vi "Mapping v10.2.0.vi"(5 "Simulate Spectra":bool, 7 "Simulate Drive":bool, 11 "Input Parameters":T7={"CCD3000 Connection"={"Comm Interface"=1, "BUS"=0, "Address"=5, "Com Port"=1}, "Drive Connection Settings"={"Objective GPIB-Port"=4, "Stage GPIB-Port"=4, "Drive Selector"=0, "Drive Velocity (V/s)"=5.0}, "ITC503 Current Values"={"ITC503 Heater"=0.0, "ITC503 Temperature"=0.0, "ITC503 P"=0.0, "ITC503 I"=0.0, "ITC503 D"=0.0, "ITC503 Setpoint"=0.0, "ITC503 Gradient"=0.0, "ITC503 Heater Auto"=FALSE, "ITC503 PID Auto"=FALSE}, "Wavelengths (nm)"=[], "Drive Current Values"={"Voltages"={"Drive X Voltage"=0.0, "Drive Y Voltage"=0.0, "Drive Z Voltage"=0.0}, "Position"={"Drive X Position"=0.0, "Drive Y Position"=0.0, "Drive Z Position"=0.0}}, "iHR Current Values"={"iHR 550 Front Entrance"=0.0, "iHR550 Side Exit"=0.0, "iHR550 Wavelength"=897.9988, "iHR550 Exit Mirror"=2, "iHR550 Grating"="1", "Grating Index"=1}, "Spectra Settings"={"Integration Time"=1.0, "Repetitions"=1, "Mapping Spectra"=TRUE}, "CCD3500 Temperature"=0.0, "Simulate Drive"=FALSE, "Simulate Spectra"=FALSE} {"CCD3500 Temperature" min=10.0 max=160.0 step=0.1 format="%.1f"; "Spectra Settings"."Repetitions" min=1 max=100 step=1; "Spectra Settings"."Integration Time" min=0.5 max=6000.0 step=1.0 format="%.1f"; "iHR Current Values"."iHR550 Exit Mirror" items=["EntranceMirror", "ExitMirror", "Front", "Side"]; "Drive Current Values"."Position"."Drive Z Position" min=-273.0 max=300000.0 step=0.0001 format="%.1f"; "Drive Current Values"."Position"."Drive Y Position" min=-273.0 max=300000.0 step=0.0001 format="%.1f"; "Drive Current Values"."Position"."Drive X Position" min=-273.0 max=300000.0 step=0.0001 format="%.1f"; "Drive Current Values"."Voltages"."Drive Z Voltage" min=-273.0 max=300000.0 step=0.0001 format="%.1f"; "Drive Current Values"."Voltages"."Drive Y Voltage" min=-273.0 max=300000.0 step=0.0001 format="%.1f"; "Drive Current Values"."Voltages"."Drive X Voltage" min=-273.0 max=300000.0 step=0.0001 format="%.1f"; "ITC503 Current Values"."ITC503 Gradient" format="%.2f"; "ITC503 Current Values"."ITC503 Setpoint" min=-273.0 max=300000.0 step=0.0001 format="%.1f"; "ITC503 Current Values"."ITC503 I" format="%_1f"; "ITC503 Current Values"."ITC503 P" format="%_1f"; "ITC503 Current Values"."ITC503 Temperature" min=0.0 max=1645.0 step=1e-05 format="%.2f"; "ITC503 Current Values"."ITC503 Heater" min=0.0 max=100.0 step=0.01 scale=0.0..100.0; "Drive Connection Settings"."Drive Velocity (V/s)" min=10.0 max=160.0 step=0.1 format="%.1f"; "Drive Connection Settings"."Drive Selector" items=["Obj.", "Stage"]; "Drive Connection Settings"."Stage GPIB-Port" min=1 max=20 step=1 format="%#.0f"; "Drive Connection Settings"."Objective GPIB-Port" min=1 max=20 step=1 format="%#.0f"; "CCD3000 Connection"."Comm Interface" items=["RS 232", "GPIB"]}) -> ()   [LabVIEW 2010]
uses:
  ESA-C/TypeDefs/ESA-C Connection Settings.ctl
  TypeDefs/Mapping Spectra Params.ctl
  TypeDefs/Mapping Drive Params.ctl
  ESA-C/TypeDefs/ESA-C Set Positions.ctl
  ESA-C/TypeDefs/ESA-C Current Values.ctl
  iHR550/TypeDefs/iHR Current Values.ctl
  ITC503/TypeDefs/ITC503 Current Values.ctl
  drivers/Horiba Spectrum One 3000V/Lib/CCD_command.llb/Comm Params.ctl
  <vilib>/Utility/miscctls.llb/LVPointTypeDef.ctl
panel:
  in  "Save Map":bool
  out "Filename":string
  out "Full Data":dbl[][](array[numeric])
  in  "CCD3000 Current Rep.":string="0/0"
  in  "CCD3500V Connection":T8={"Comm Interface"=1, "BUS"=0, "Address"=5, "Com Port"=0}
  out "Live Data":dbl[][](array[numeric])
  in  "ITC503 Current Values":T3 {"ITC503 Gradient" format="%.2f"; "ITC503 Setpoint" min=-273.0 max=300000.0 step=0.0001 format="%.1f"; "ITC503 I" format="%_1f"; "ITC503 P" format="%_1f"; "ITC503 Temperature" min=0.0 max=1645.0 step=1e-05 format="%.2f"; "ITC503 Heater" min=0.0 max=100.0 step=0.01 scale=0.0..100.0}
  in  "iHR Current Values":T5={"iHR 550 Front Entrance"=0.0, "iHR550 Side Exit"=0.0, "iHR550 Wavelength"=897.9988, "iHR550 Exit Mirror"=2, "iHR550 Grating"="1", "Grating Index"=1} {"iHR550 Exit Mirror" items=["EntranceMirror", "ExitMirror", "Front", "Side"]}
  in  "CCD3500 Temperature":dbl caption="Temp. (°C)" min=10.0 max=160.0 step=0.1 format="%.1f"
  in  "Wavelengths (nm)":dbl[](array[numeric])
  in  "Spectra Params":T6={"Integration Time"=10.0, "Repetitions"=10, "Mapping Spectra"=TRUE} {"Repetitions" min=1 max=100 step=1; "Integration Time" min=0.5 max=6000.0 step=1.0 format="%.1f"}
  in  "Drive Settings":T2={"Objective GPIB-Port"=4, "Stage GPIB-Port"=4, "Drive Selector"=0, "Drive Velocity (V/s)"=5.0} {"Drive Velocity (V/s)" min=10.0 max=160.0 step=0.1 format="%.1f"; "Drive Selector" items=["Obj.", "Stage"]; "Stage GPIB-Port" min=1 max=20 step=1 format="%#.0f"; "Objective GPIB-Port" min=1 max=20 step=1 format="%#.0f"}
  out "Current Position":T4 {"Position"."Drive Z Position" min=-273.0 max=300000.0 step=0.0001 format="%.1f"; "Position"."Drive Y Position" min=-273.0 max=300000.0 step=0.0001 format="%.1f"; "Position"."Drive X Position" min=-273.0 max=300000.0 step=0.0001 format="%.1f"; "Voltages"."Drive Z Voltage" min=-273.0 max=300000.0 step=0.0001 format="%.1f"; "Voltages"."Drive Y Voltage" min=-273.0 max=300000.0 step=0.0001 format="%.1f"; "Voltages"."Drive X Voltage" min=-273.0 max=300000.0 step=0.0001 format="%.1f"}
  out "Target Position":T9={"Drive X Set"=10.0, "Drive Y Set"=10.0, "Drive Z Set"=10.0} {"Drive X Set" min=10.0 max=160.0 step=0.1 format="%.1f"; "Drive Z Set" min=10.0 max=160.0 step=0.1 format="%.1f"; "Drive Y Set" min=10.0 max=160.0 step=0.1 format="%.1f"}
  out "Progress":u8(slide) max=10 scale=0.0..100.0
  out "Objective Running":bool caption="Obj."
  out "CCD Running":bool caption="CCD"
  in  "Z Position":dbl caption="Z (µm)" min=0.0 max=100.0 step=0.1 format="%.1f"
  in  "Mapping Params":T10={"X Start Position"=0.0, "X Stop Position"=10.0, "Y Start Position"=0.0, "Y Stop Position"=10.0, "Step Size"=1.0} {"Step Size" min=0.1 max=30.0 step=0.1 format="%.1f"; "Y Stop Position" min=0.0 max=30.0 step=0.1 format="%.1f"; "Y Start Position" min=0.0 max=30.0 step=0.1 format="%.1f"; "X Stop Position" min=0.0 max=30.0 step=0.1 format="%.1f"; "X Start Position" min=0.0 max=30.0 step=0.1 format="%.1f"}
  in  "Exit":bool
  out "Measuring":bool
  in  "Start":bool
  # "Spectral"
  # "Spectral / Video Mapping"
  # "Parameters"
  # "GPIB"
  # "Status"
  # "Active"
  # "Target"
  # "Current"
  # "Mapping"
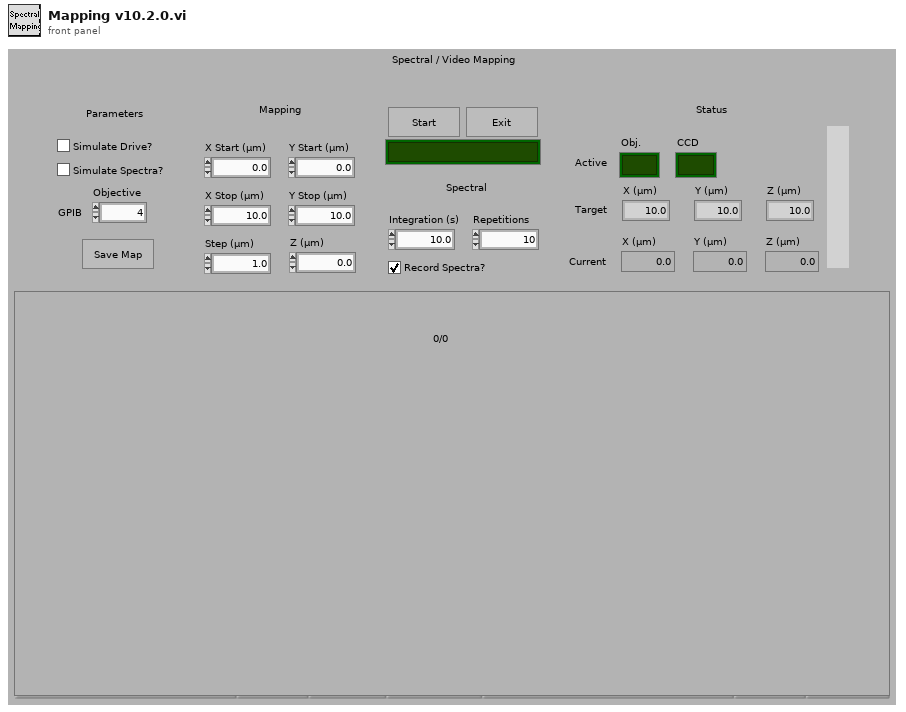
[diagram p1: front panel]
types:
  T1 = typedef "Comm Params.ctl" = cluster{"Comm Interface":u16, "BUS":i16, "Address":i16, "Com Port":i32}
  T2 = typedef "ESA-C Connection Settings.ctl" = cluster{"Objective GPIB-Port":i32, "Stage GPIB-Port":i32, "Drive Selector":u16, "Drive Velocity (V/s)":dbl}
  T3 = typedef "ITC503 Current Values.ctl" = cluster{"ITC503 Heater":dbl, "ITC503 Temperature":dbl, "ITC503 P":dbl, "ITC503 I":dbl, "ITC503 D":dbl, "ITC503 Setpoint":dbl, "ITC503 Gradient":dbl, "ITC503 Heater Auto":bool, "ITC503 PID Auto":bool}
  T4 = typedef "ESA-C Current Values.ctl" = cluster{"Voltages":cluster{"Drive X Voltage":dbl, "Drive Y Voltage":dbl, "Drive Z Voltage":dbl}, "Position":cluster{"Drive X Position":dbl, "Drive Y Position":dbl, "Drive Z Position":dbl}}
  T5 = typedef "iHR Current Values.ctl" = cluster{"iHR 550 Front Entrance":dbl, "iHR550 Side Exit":dbl, "iHR550 Wavelength":dbl, "iHR550 Exit Mirror":i32, "iHR550 Grating":string, "Grating Index":i32}
  T6 = typedef "Mapping Spectra Params.ctl" = cluster{"Integration Time":dbl, "Repetitions":u16, "Mapping Spectra":bool}
  T7 = cluster{"CCD3000 Connection":T1, "Drive Connection Settings":T2, "ITC503 Current Values":T3, "Wavelengths (nm)":dbl[], "Drive Current Values":T4, "iHR Current Values":T5, "Spectra Settings":T6, "CCD3500 Temperature":dbl, "Simulate Drive":bool, "Simulate Spectra":bool}
  T8 = cluster{"Comm Interface":u16, "BUS":i16, "Address":i16, "Com Port":i32}
  T9 = typedef "ESA-C Set Positions.ctl" = cluster{"Drive X Set":dbl, "Drive Y Set":dbl, "Drive Z Set":dbl}
  T10 = typedef "Mapping Drive Params.ctl" = cluster{"X Start Position":dbl, "X Stop Position":dbl, "Y Start Position":dbl, "Y Stop Position":dbl, "Step Size":dbl}
  T11 = cluster{"CCD3000 Connection":T1, "Drive Connection Settings":T2, "ITC503 Current Values":T3, "Wavelengths (nm)":dbl[], "Drive Current Values":T4, "iHR Current Values":T5, "Spectra Settings":T6, "CCD3500 Temperature":dbl, "Simulate Drive 2":bool, "Simulate Spectra 2":bool}
  T12 = typedef "LVPointTypeDef.ctl" = cluster{"Horizontal":i16, "Vertical":i16}
  T13 = typedef "NPC3SG Set Positions.ctl" = cluster{"Drive X Set":dbl, "Drive Y Set":dbl, "Drive Z Set":dbl}
  T14 = cluster{"Intensities":dbl[], "Wavelengths":dbl[]}[]
  T15 = cluster{"Intensities":dbl[], "Wavelengths":dbl[]}
  T16 = enum32{"invalid app kind", "Development System", "Run Time System", "Student Edition", "Embedded LabVIEW", "Evaluation", "Custom"}
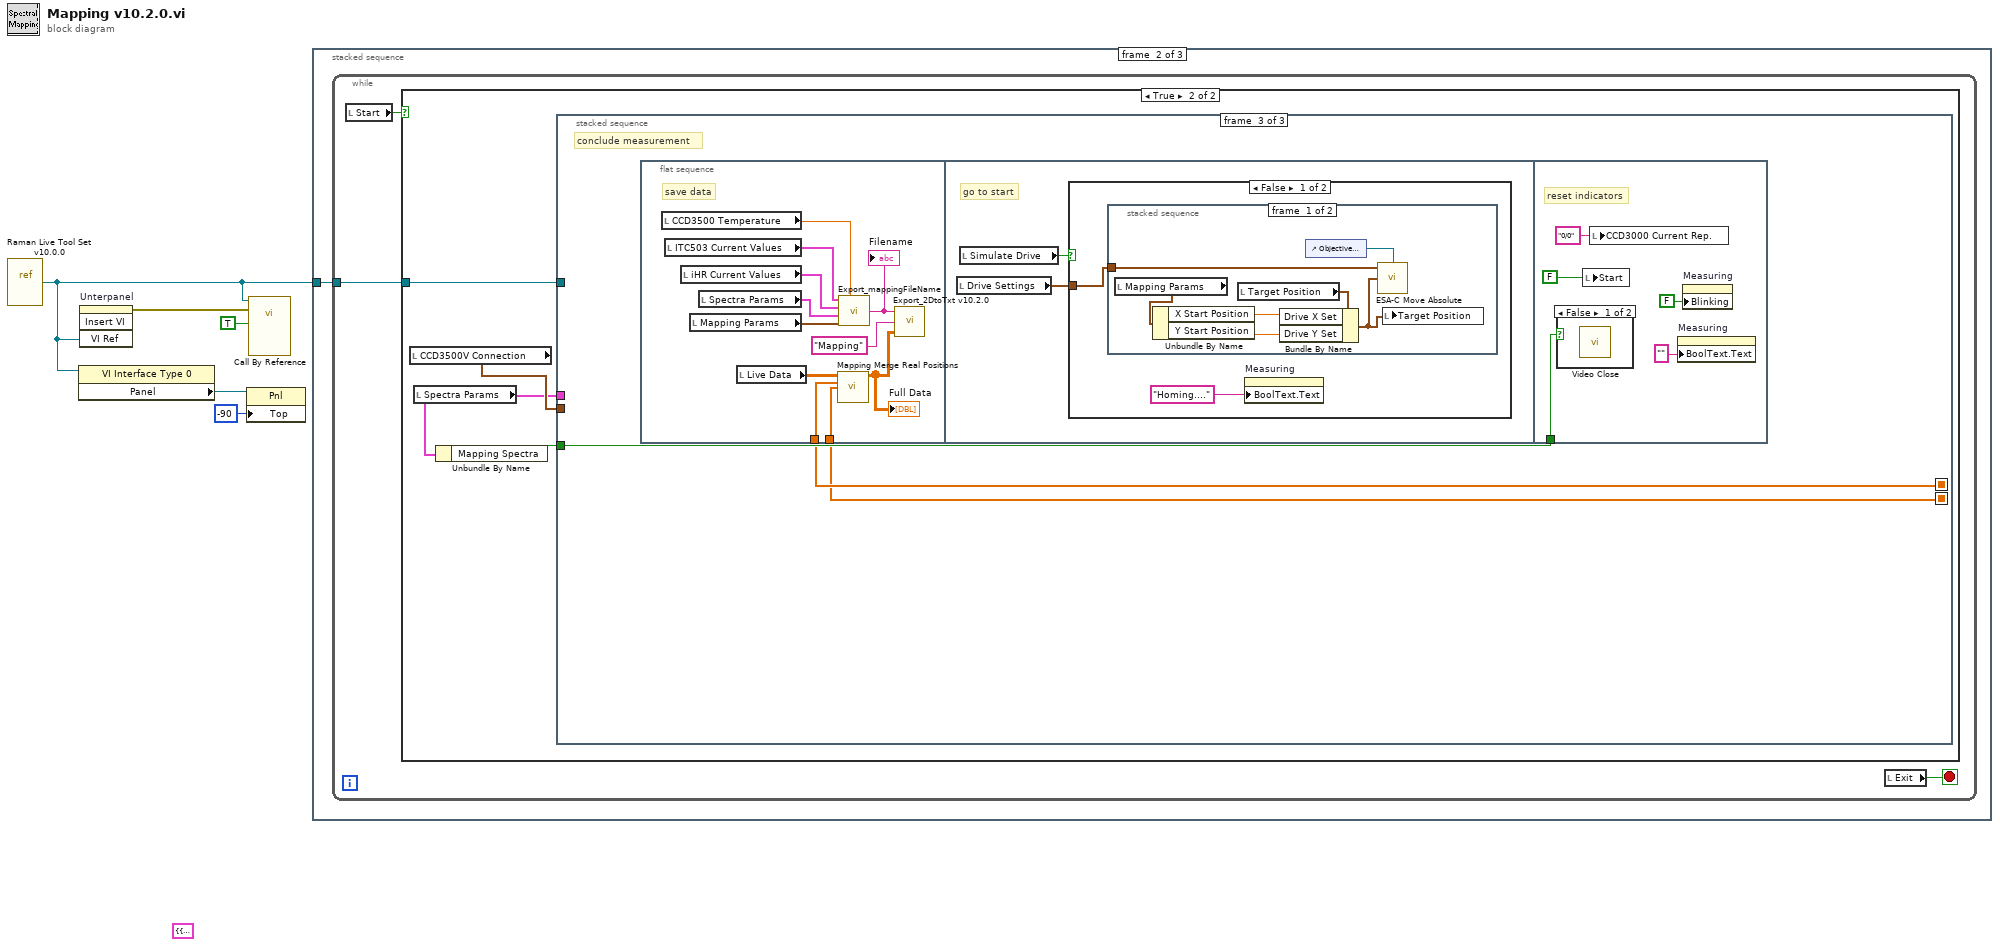
[diagram p0: block diagram]
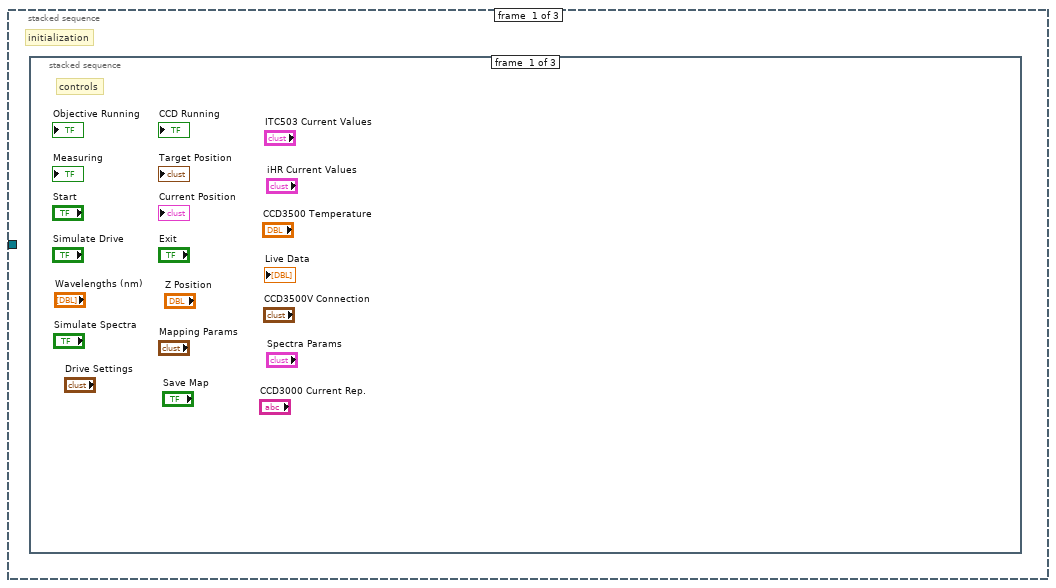
[diagram p2: hidden frame]
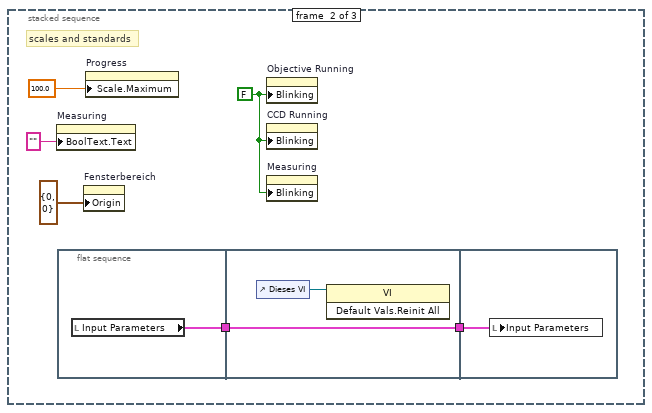
[diagram p3: hidden frame]
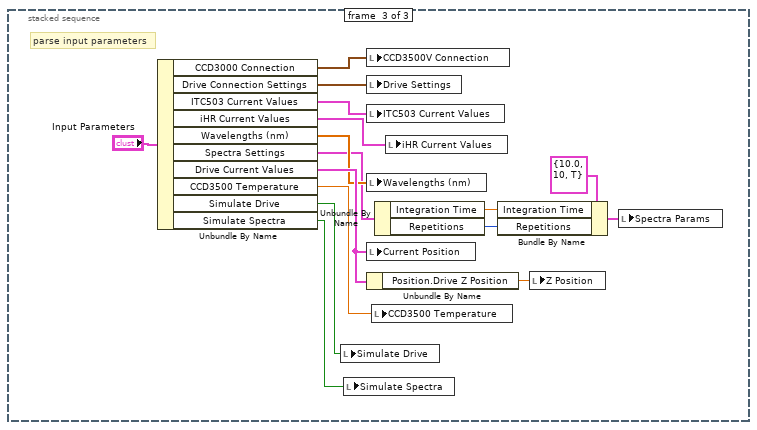
[diagram p4: hidden frame]
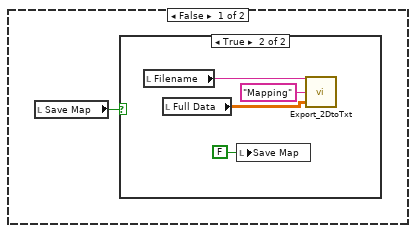
[diagram p5: hidden frame]
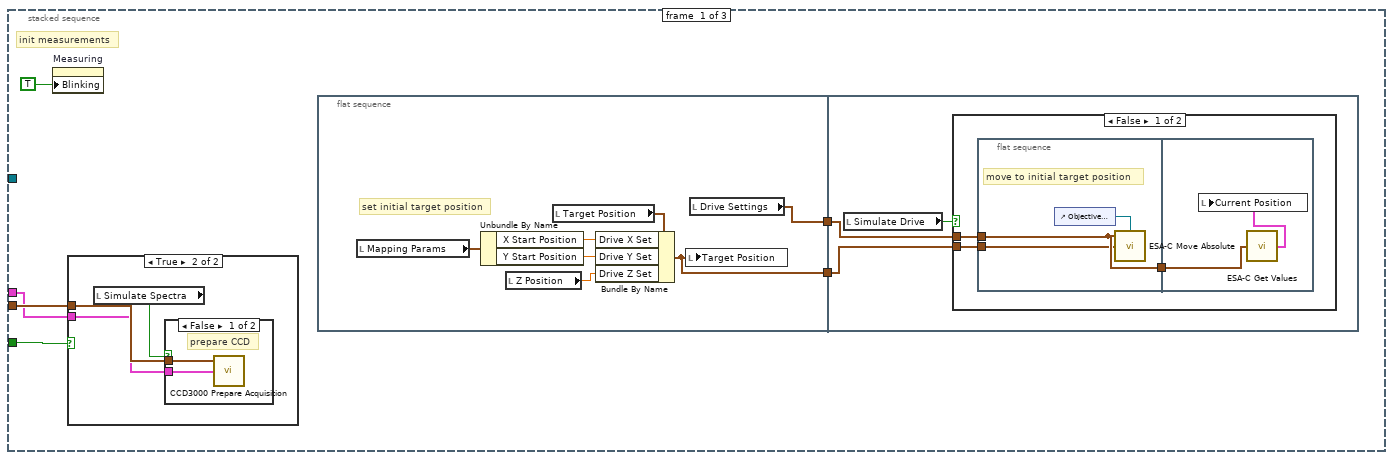
[diagram p7: hidden frame]
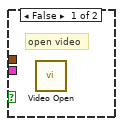
[diagram p9: hidden frame]
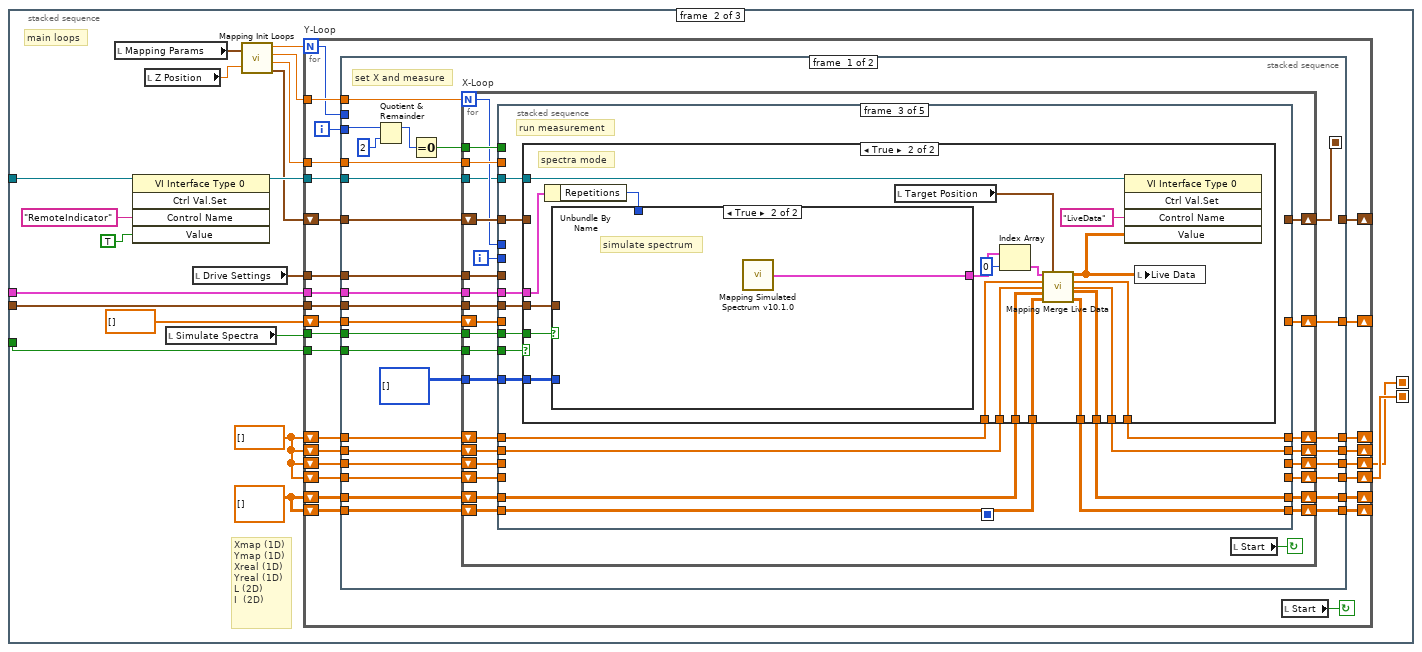
[diagram p11: hidden frame]
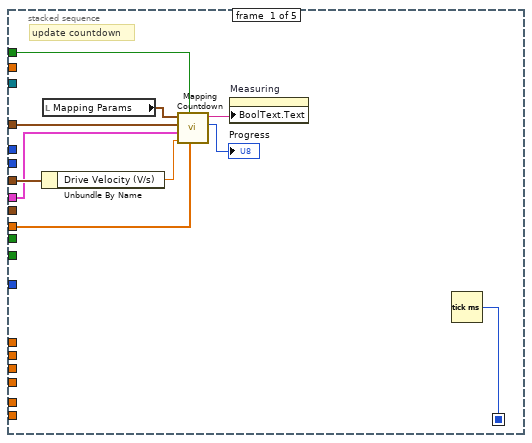
[diagram p12: hidden frame]
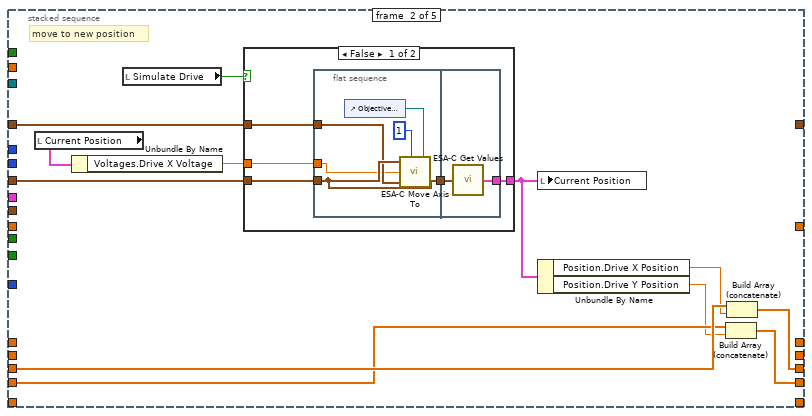
[diagram p13: hidden frame]
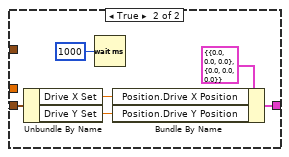
[diagram p14: hidden frame]
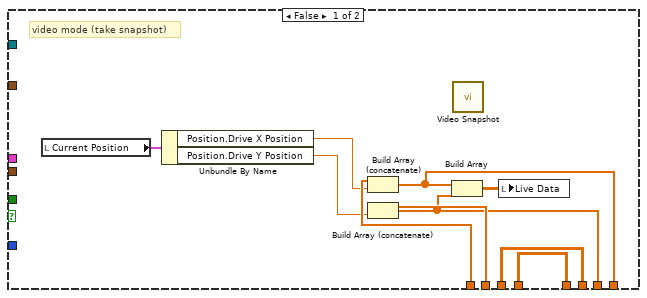
[diagram p15: hidden frame]
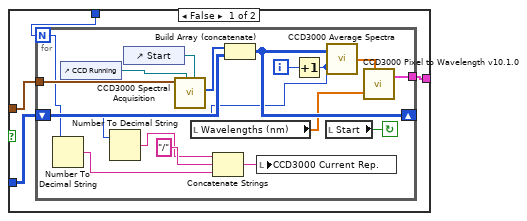
[diagram p16: hidden frame]
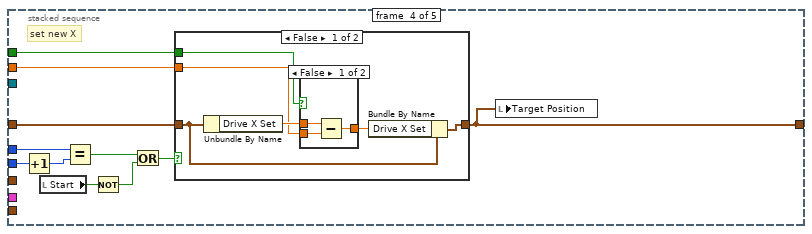
[diagram p17: hidden frame]
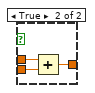
[diagram p18: hidden frame]
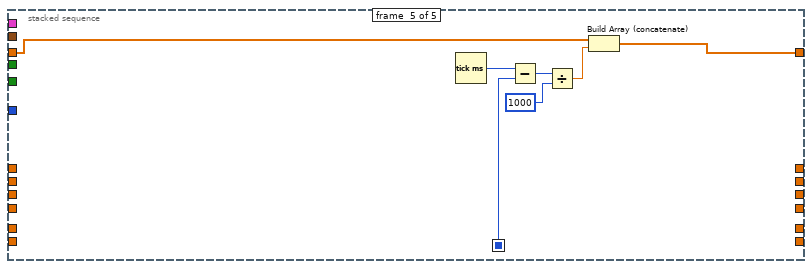
[diagram p20: hidden frame]
diagram:
  (unwired) T11 {"CCD3000 Connection"={"Comm Interface"=1, "BUS"=0, "Address"=5, "Com Port"=1}, "Drive Connection Settings"={"Objective GPIB-Port"=4, "Stage GPIB-Port"=4, "Drive Selector"=0, "Drive Velocity (V/s)"=5.0}, "ITC503 Current Values"={"ITC503 Heater"=0.0, "ITC503 Temperature"=0.0, "ITC503 P"=0.0, "ITC503 I"=0.0, "ITC503 D"=0.0, "ITC503 Setpoint"=0.0, "ITC503 Gradient"=0.0, "ITC503 Heater Auto"=FALSE, "ITC503 PID Auto"=FALSE}, "Wavelengths (nm)"=[], "Drive Current Values"={"Voltages"={"Drive X Voltage"=0.0, "Drive Y Voltage"=0.0, "Drive Z Voltage"=0.0}, "Position"={"Drive X Position"=0.0, "Drive Y Position"=0.0, "Drive Z Position"=0.0}}, "iHR Current Values"={"iHR 550 Front Entrance"=0.0, "iHR550 Side Exit"=0.0, "iHR550 Wavelength"=897.9988, "iHR550 Exit Mirror"=2, "iHR550 Grating"="1", "Grating Index"=1}, "Spectra Settings"={"Integration Time"=1.0, "Repetitions"=1, "Mapping Spectra"=TRUE}, "CCD3500 Temperature"=0.0, "Simulate Drive 2"=FALSE, "Simulate Spectra 2"=FALSE} ("Input Parameters")
  n1 = vi-ref "Raman Live Tool Set v10.0.0.vi"() -> (w3:refnum<vi>)
  n2 = property class="VI Interface Type 0"(reference=w3) -> ("Panel"=w2:refnum<vi>)  [unwired: 1 in, 2 out]
  n3 = invoke on="Unterpanel" class="Unterpanel" method="Insert VI"("VI Ref"=w3) -> (error out=w5:errorcluster)  [unwired: 3 in, 3 out]
  n4 = property class="Pnl"(reference=w2, "Top"=-90 ("Position:Oben")) -> ()  [unwired: 1 in, 2 out]
  n5 = call-by-ref "?"(reference=w3, error in=w5, "RemoteIndicator"=TRUE) -> ()  [unwired: 3 in, 2 out]
  n6 = stacked-sequence {
    tunnel: w3 -> [_ w32 w379]
    frame #0 {
      # "initialization"
      n7 = stacked-sequence {
        frame #0 {
          # "controls"
        }
        frame #1 {
          w9 = FALSE ("Blinkend")
          # "scales and standards"
          n8 = property on="Measuring" class="Bool (strict)"("BoolText.Text"="" ("Boolescher Text.Text")) -> ()  [unwired: 2 in, 2 out]
          n9 = flat-sequence {
            tunnel: [w12] -> w6
            tunnel: [w13] -> w7
            tunnel: w6 -> [w13]
            tunnel: w7 -> [w15]
            frame #0 {
              n10 = local read "Input Parameters"() -> (w12:T7)
            }
            frame #1 {
              n11 = control-ref of="Dieses VI"() -> (w14:refnum<vi>)
              n12 = invoke class="VI" method="Default Vals.Reinit All"(reference=w14) -> ()  [unwired: 2 in, 3 out]
            }
            frame #2 {
              n13 = local write "Input Parameters"(w15) -> ()
            }
          }
          n14 = property on="Fensterbereich" class="Pane"("Origin"=T12 {"Horizontal"=0, "Vertical"=0}) -> ()  [unwired: 2 in, 2 out]
          n15 = property on="Progress" class="Slide (strict)"("Scale.Maximum"=100.0 ("Skalierung.Bereich:Maximum")) -> ()  [unwired: 2 in, 2 out]
          n16 = property on="Objective Running" class="Bool (strict)"("Blinking"=w9) -> ()  [unwired: 2 in, 2 out]
          n17 = property on="CCD Running" class="Bool (strict)"("Blinking"=w9) -> ()  [unwired: 2 in, 2 out]
          n18 = property on="Measuring" class="Bool (strict)"("Blinking"=w9) -> ()  [unwired: 2 in, 2 out]
        }
        frame #2 {
          # "parse input parameters"
          n19 = Unbundle By Name("Input Parameters") -> ("CCD3000 Connection"=w28:T1, "Drive Connection Settings"=w29:T2, "ITC503 Current Values"=w30:T3, "iHR Current Values"=w19:T5, "Wavelengths (nm)"=w27:dbl[], "Spectra Settings"=w25:T6, "Drive Current Values"=w31:T4, "CCD3500 Temperature"=w20:dbl, "Simulate Drive"=w17:bool, "Simulate Spectra"=w16:bool)
          n20 = local write "Simulate Drive"(w17) -> ()
          n21 = local write "Simulate Spectra"(w16) -> ()
          n22 = local write "CCD3500V Connection"(w28) -> ()
          n23 = local write "Drive Settings"(w29) -> ()
          n24 = local write "ITC503 Current Values"(w30) -> ()
          n25 = local write "Wavelengths (nm)"(w27) -> ()
          n26 = local write "Current Position"(w31) -> ()
          n27 = Unbundle By Name(w31) -> ("Position.Drive Z Position"=w26:dbl)
          n28 = local write "CCD3500 Temperature"(w20) -> ()
          n29 = Unbundle By Name(w25) -> ("Integration Time"=w23:dbl, "Repetitions"=w22:u16)
          n30 = local write "iHR Current Values"(w19) -> ()
          n31 = Bundle By Name(cluster=T6 {"Integration Time"=10.0, "Repetitions"=10, "Mapping Spectra"=TRUE} ("Mapping Spectra Settings"), "Integration Time"=w23, "Repetitions"=w22) -> (w21:T6)
          n32 = local write "Z Position"(w26) -> ()
          n33 = local write "Spectra Params"(w21) -> ()
        }
      }
    }
    frame #1 {
      n34 = while {
        tunnel: w32 -> [w35]
        stop <- w34 stop-if-true
        n35 = local read "Start"() -> (w33:bool)
        n36 = case shown="True" w33 {
          tunnel: w35 -> [_ w44]
          frame False {
            n37 = local read "Save Map"() -> (w36:bool)
            n38 = case shown="True" w36 {
              frame False {
              }
              frame True {
                n39 = local read "Filename"() -> (w39:string)
                n40 = local read "Full Data"() -> (w37:dbl[][])
                n41 = local write "Save Map"(FALSE ("Save Map")) -> ()
                n42 = call "Export_2DtoTxt.vi"("Data (2D)"=w37, "Export Type"="Mapping", "Filename"=w39) -> ()  [unwired: 3 in]
              }
            }
          }
          frame True {
            n43 = local read "CCD3500V Connection"() -> (w42:T8)
            n44 = local read "Spectra Params"() -> (w41:T6)
            n45 = Unbundle By Name(w41) -> ("Mapping Spectra"=w43:bool)
            n46 = stacked-sequence {
              seq-local: [_ w74 _] -> [_ _ w348]
              seq-local: [_ w75 _] -> [_ _ w347]
              tunnel: w44 -> [_ w85 _]
              tunnel: w43 -> [w49 w84 w349]
              tunnel: w41 -> [w47 w82 _]
              tunnel: w42 -> [w48 w81 _]
              frame #0 {
                # "init measurements"
                n47 = property on="Measuring" class="Bool (strict)"("Blinking"=TRUE ("Blinkend")) -> ()  [unwired: 2 in, 2 out]
                n48 = case shown="True" w49 {
                  tunnel: w48 -> [_ w71]
                  tunnel: w47 -> [_ w70]
                  frame False {
                    # "open video"
                    n49 = call "Video Open.vi"() -> ()  [unwired: 11 in, 1 out]
                  }
                  frame True {
                    n50 = local read "Simulate Spectra"() -> (w69:bool)
                    n51 = case shown="False" w69 {
                      tunnel: w71 -> [w73 _]
                      tunnel: w70 -> [w72 _]
                      frame False {
                        # "prepare CCD"
                        n52 = call "CCD3000 Prepare Acquisition.vi"("Mapping Spectra Settings"=w72, "Comm Params"=w73) -> ()  [unwired: 4 in]
                      }
                      frame True {
                      }
                    }
                  }
                }
                n53 = flat-sequence {
                  tunnel: [w52] -> w46
                  tunnel: [w51] -> w45
                  tunnel: w46 -> [w58]
                  tunnel: w45 -> [w59]
                  frame #0 {
                    # "set initial target position"
                    n54 = local read "Mapping Params"() -> (w57:T10)
                    n55 = Unbundle By Name(w57) -> ("X Start Position"=w55:dbl, "Y Start Position"=w54:dbl)
                    n56 = local read "Z Position"() -> (w53:dbl)
                    n57 = local read "Target Position"() -> (w56:T9)
                    n58 = Bundle By Name(cluster=w56, "Drive X Set"=w55, "Drive Y Set"=w54, "Drive Z Set"=w53) -> (w52:T9)
                    n59 = local write "Target Position"(w52) -> ()
                    n60 = local read "Drive Settings"() -> (w51:T2)
                  }
                  frame #1 {
                    n61 = local read "Simulate Drive"() -> (w60:bool)
                    n62 = case shown="False" w60 {
                      tunnel: w59 -> [w63 _]
                      tunnel: w58 -> [w61 _]
                      frame False {
                        n63 = flat-sequence {
                          tunnel: w63 -> [w65]
                          tunnel: [w65] -> w62
                          tunnel: w61 -> [w64]
                          tunnel: w62 -> [w68]
                          frame #0 {
                            # "move to initial target position"
                            n64 = control-ref of="Objective Running"() -> (w66:refnum<vi>)
                            n65 = call "ESA-C Move Absolute.vi"("Running"=w66, "Drive New Abs. Positions"=w64, "Drive Connection Settings"=w65) -> ()  [unwired: 2 in]
                          }
                          frame #1 {
                            n66 = call "ESA-C Get Values.vi"("Drive Connection Settings"=w68) -> ("Drive Current Values"=w67:T4)
                            n67 = local write "Current Position"(w67) -> ()
                          }
                        }
                      }
                      frame True {
                      }
                    }
                  }
                }
              }
              frame #1 {
                w93 = dbl[][] []
                w76 = dbl[] []
                # "main loops"
                # "Xmap (1D)\nYmap (1D)\nXreal (1D)\nYreal (1D)\nL (2D)\nI  (2D)"
                n68 = local read "Mapping Params"() -> (w79:T10)
                n69 = invoke class="VI Interface Type 0" method="Ctrl Val.Set"(reference=w85, "Control Name"="RemoteIndicator" ("Elementname"), "Value"=TRUE) -> (reference out=w87:refnum<vi>)  [unwired: 2 in, 4 out]
                n70 = local read "Z Position"() -> (w78:dbl)
                n71 = local read "Simulate Spectra"() -> (w77:bool)
                n72 = local read "Drive Settings"() -> (w80:T2)
                n73 = call "Mapping Init Loops.vi"("Z Position"=w78, "Mapping Params"=w79) -> ("Start Positions"=w86:T13, "Step Size"=w88:dbl, "X Steps"=w89:dbl, "Y Steps"=w90:dbl)
                n74 = for "Y-Loop" {
                  N: w90 -> [w106]
                  tunnel: w89 -> [w119]
                  tunnel: w88 -> [w118]
                  shift-right: [w104] -> _
                  shift-left: w86 -> [w105]
                  shift-right: [w110] -> _
                  shift-left: w93 -> [w114]
                  shift-right: [w111] -> _
                  shift-left: w93 -> [w115]
                  shift-right: [w113] -> _
                  shift-left: w76 -> [w117]
                  shift-right: [w112] -> _
                  shift-left: w76 -> [w116]
                  tunnel: w87 -> [w108]
                  tunnel: w77 -> [w107]
                  tunnel: w80 -> [w103]
                  tunnel: w84 -> [w102]
                  tunnel: w82 -> [w101]
                  shift-right: [w99] -> _
                  shift-left: dbl[] [] -> [w100]
                  tunnel: w81 -> [w98]
                  shift-right: [w95] -> w75
                  shift-left: w76 -> [w96]
                  shift-right: [w94] -> w74
                  shift-left: w76 -> [w97]
                  i -> [w109]
                  stop <- w120 continue-if-true
                  n75 = stacked-sequence {
                    seq-local: [w133 _] -> [_ w323]
                    tunnel: w119 -> [w149 _]
                    tunnel: w118 -> [w148 w324]
                    tunnel: w117 -> [w147 _]
                    tunnel: w116 -> [w146 _]
                    tunnel: w115 -> [w145 _]
                    tunnel: w114 -> [w144 _]
                    tunnel: [w143 _] -> w113
                    tunnel: [w142 _] -> w112
                    tunnel: [w141 _] -> w111
                    tunnel: [w140 _] -> w110
                    tunnel: w109 -> [w137 w327]
                    tunnel: w108 -> [w135 _]
                    tunnel: w107 -> [w134 _]
                    tunnel: w106 -> [_ w325]
                    tunnel: w105 -> [w132 _]
                    tunnel: [_ w321] -> w104
                    tunnel: w103 -> [w131 w322]
                    tunnel: w102 -> [w130 _]
                    tunnel: w101 -> [w129 _]
                    tunnel: w100 -> [w128 _]
                    tunnel: [w127 _] -> w99
                    tunnel: w98 -> [w126 _]
                    tunnel: w97 -> [w124 _]
                    tunnel: w96 -> [w123 _]
                    tunnel: [w122 _] -> w95
                    tunnel: [w121 _] -> w94
                    frame #0 {
                      # "set X and measure"
                      n76 = Quotient & Remainder(x=w137, y=2) -> (x-y*floor(x/y)=w138:i32)  [unwired: 1 out]
                      n77 = Equal To 0?(x=w138) -> (x = 0?=w136:bool)
                      n78 = for "X-Loop" {
                        N: w149 -> [w163]
                        tunnel: w148 -> [w175]
                        shift-right: [w174] -> w133
                        shift-left: w132 -> [w176]
                        shift-right: [w169] -> w143
                        shift-left: w147 -> [w173]
                        shift-right: [w168] -> w142
                        shift-left: w146 -> [w172]
                        shift-right: [w166] -> w141
                        shift-left: w145 -> [w171]
                        shift-right: [w167] -> w140
                        shift-left: w144 -> [w170]
                        tunnel: w136 -> [w165]
                        tunnel: w135 -> [w162]
                        tunnel: w134 -> [w161]
                        tunnel: w131 -> [w160]
                        tunnel: w130 -> [w159]
                        tunnel: w129 -> [w158]
                        shift-right: [w157] -> w127
                        shift-left: w128 -> [w156]
                        tunnel: w126 -> [w155]
                        tunnel: u16[][] [] -> [w154]
                        shift-right: [w150] -> w121
                        shift-left: w124 -> [w153]
                        shift-right: [w151] -> w122
                        shift-left: w123 -> [w152]
                        i -> [w164]
                        stop <- w177 continue-if-true
                        n79 = stacked-sequence {
                          seq-local: [w178 _ _ _ _] -> [_ _ _ _ w312]
                          tunnel: w176 -> [w183 w199 w232 w292 _]
                          tunnel: w175 -> [_ _ _ w290 _]
                          tunnel: [_ _ _ w289 _] -> w174
                          tunnel: w173 -> [_ _ w231 _ _]
                          tunnel: w172 -> [_ _ w230 _ _]
                          tunnel: w171 -> [_ _ w228 _ _]
                          tunnel: w170 -> [_ _ w229 _ _]
                          tunnel: [_ _ w227 _ _] -> w169
                          tunnel: [_ _ w226 _ _] -> w168
                          tunnel: [_ _ w225 _ _] -> w167
                          tunnel: [_ _ w224 _ _] -> w166
                          tunnel: w165 -> [w184 _ _ w291 _]
                          tunnel: w164 -> [_ _ _ w295 _]
                          tunnel: w163 -> [_ _ _ w293 _]
                          tunnel: w162 -> [_ _ w223 _ _]
                          tunnel: w161 -> [_ _ w222 _ _]
                          tunnel: w160 -> [w181 w197 _ _ _]
                          tunnel: w159 -> [_ _ w221 _ _]
                          tunnel: w158 -> [w180 _ w219 _ _]
                          tunnel: [_ _ _ _ w309] -> w157
                          tunnel: w156 -> [w179 _ _ _ w311]
                          tunnel: w155 -> [_ _ w220 _ _]
                          tunnel: w154 -> [_ _ w218 _ _]
                          tunnel: w153 -> [_ w193 _ _ _]
                          tunnel: w152 -> [_ w192 _ _ _]
                          tunnel: [_ w189 _ _ _] -> w151
                          tunnel: [_ w188 _ _ _] -> w150
                          frame #0 {
                            # "update countdown"
                            n80 = Unbundle By Name(w181) -> ("Drive Velocity (V/s)"=w182:dbl)
                            n81 = local read "Mapping Params"() -> (w187:T10)
                            n82 = call "Mapping Countdown.vi"("Execution Times (s)"=w179, "Forward?"=w184, "Drive Velocity"=w182, "Mapping Spectra Settings"=w180, "Drive New Abs. Positions"=w183, "Mapping Drive Parameters"=w187) -> ("Progress"=→"Progress":i16, "Time String"=w185:string)  [unwired: 4 in]
                            n83 = property on="Measuring" class="Bool (strict)"("BoolText.Text"=w185) -> ()  [unwired: 2 in, 2 out]
                            n84 = Tick Count (ms)() -> (millisecond timer value=w178:u32)
                          }
                          frame #1 {
                            # "move to new position"
                            n85 = local read "Current Position"() -> (w196:T4)
                            n86 = Unbundle By Name(w196) -> ("Voltages.Drive X Voltage"=w195:dbl)
                            n87 = local read "Simulate Drive"() -> (w198:bool)
                            n88 = case shown="False" w198 {
                              tunnel: w199 -> [w203 w216]
                              tunnel: [w202 w213] -> w194
                              tunnel: w197 -> [w201 _]
                              tunnel: w195 -> [w200 _]
                              frame False {
                                n89 = flat-sequence {
                                tunnel: w203 -> [w208]
                                tunnel: [w209] -> w204
                                tunnel: w201 -> [w209]
                                tunnel: w200 -> [w205]
                                tunnel: w204 -> [w211]
                                tunnel: [w210] -> w202
                                frame #0 {
                                n90 = control-ref of="Objective Running"() -> (w206:refnum<vi>)
                                n91 = call "ESA-C Move Axis To.vi"("Drive Connection Settings"=w209, "Axis"=1, "Current Voltage (V)"=w205, "Drive New Abs. Positions"=w208, "Running"=w206) -> ()  [unwired: 2 in]
                                }
                                frame #1 {
                                n92 = call "ESA-C Get Values.vi"("Drive Connection Settings"=w211) -> ("Drive Current Values"=w210:T4)
                                }
                                }
                              }
                              frame True {
                                n93 = Unbundle By Name(w216) -> ("Drive X Set"=w217:dbl, "Drive Y Set"=w214:dbl)
                                n94 = Wait (ms)(milliseconds to wait=u32 1000 ("Zu wartende ms")) -> ()  [unwired: 1 out]
                                n95 = Bundle By Name(cluster=T4 {"Voltages"={"Drive X Voltage"=0.0, "Drive Y Voltage"=0.0, "Drive Z Voltage"=0.0}, "Position"={"Drive X Position"=0.0, "Drive Y Position"=0.0, "Drive Z Position"=0.0}} ("Drive Current Values"), "Position.Drive X Position"=w217, "Position.Drive Y Position"=w214) -> (w213:T4)
                              }
                            }
                            n96 = local write "Current Position"(w194) -> ()
                            n97 = Unbundle By Name(w194) -> ("Position.Drive X Position"=w191:dbl, "Position.Drive Y Position"=w190:dbl)
                            n98 = Build Array (concatenate)(w192, w190) -> (w189:dbl[])
                            n99 = Build Array (concatenate)(w193, w191) -> (w188:dbl[])
                          }
                          frame #2 {
                            # "run measurement"
                            n100 = case shown="True" w221 {
                              tunnel: w232 -> [_ _]
                              tunnel: w231 -> [w239 w259]
                              tunnel: w230 -> [w238 w258]
                              tunnel: w229 -> [w241 w256]
                              tunnel: w228 -> [w242 w257]
                              tunnel: [w236 w253] -> w227
                              tunnel: [w237 w252] -> w226
                              tunnel: [w241 w255] -> w225
                              tunnel: [w242 w254] -> w224
                              tunnel: w223 -> [_ w261]
                              tunnel: w222 -> [_ w260]
                              tunnel: w220 -> [_ w249]
                              tunnel: w219 -> [_ w248]
                              tunnel: w218 -> [_ w246]
                              frame False {
                                # "video mode (take snapshot)"
                                n101 = local read "Current Position"() -> (w240:T4)
                                n102 = Unbundle By Name(w240) -> ("Position.Drive X Position"=w235:dbl, "Position.Drive Y Position"=w234:dbl)
                                n103 = Build Array (concatenate)(w239, w235) -> (w236:dbl[])
                                n104 = Build Array (concatenate)(w238, w234) -> (w237:dbl[])
                                n105 = Build Array(w236, w237) -> (w233:dbl[][])
                                n106 = call "Video Snapshot.vi"() -> ()  [unwired: 11 in, 1 out]
                                n107 = local write "Live Data"(w233) -> ()
                              }
                              frame True {
                                # "spectra mode"
                                n108 = Unbundle By Name(w248) -> ("Repetitions"=w247:u16)
                                n109 = case shown="True" w260 {
                                tunnel: [w265 w284] -> w245
                                tunnel: w249 -> [w266 _]
                                tunnel: w247 -> [w264 _]
                                tunnel: w246 -> [w263 _]
                                frame False {
                                n110 = for {
                                N: w264 -> [w268]
                                shift-right: [w280] -> _
                                shift-left: w263 -> [w281]
                                tunnel: [w278] -> w265
                                tunnel: w266 -> [w276]
                                i -> [w283]
                                stop <- w275 continue-if-true
                                n111 = Number To Decimal String(number=w268) -> (decimal integer string=w271:string)  [unwired: 1 in]
                                n112 = control-ref of="CCD Running"() -> (w274:refnum<vi>)
                                n113 = control-ref of="Start"() -> (w273:refnum<vi>)
                                n114 = call "CCD3000 Spectral Acquisition.vi"("Acquire"=w273, "Running"=w274, "Comm Params"=w276) -> ("Raw-Spectrum"=w282:u16[])  [unwired: 6 in, 2 out]
                                n115 = local read "Wavelengths (nm)"() -> (w277:dbl[])
                                n116 = Build Array (concatenate)(w282, w281) -> (w280:u16[][])
                                n117 = Increment(x=w283) -> (x+1=w267:i32)
                                n118 = Number To Decimal String(number=w267) -> (decimal integer string=w270:string)  [unwired: 1 in]
                                n119 = Concatenate Strings(w270, "/" ("string"), w271) -> (w269:string)
                                n120 = local write "CCD3000 Current Rep."(w269) -> ()
                                n121 = local read "Start"() -> (w275:bool)
                                n122 = call "CCD3000 Average Spectra.vi"("Repetitions"=w267, "Raw Spectra"=w280) -> ("Raw Spectrum"=w279:dbl[])
                                n123 = call "CCD3000 Pixel to Wavelength v10.1.0.vi"("Wavelengths (nm)"=w277, "Raw Spectrum"=w279) -> ("Spectrum-Cluster"=w278:T14)  [unwired: 1 out]
                                }
                                }
                                frame True {
                                # "simulate spectrum"
                                n124 = call "Mapping Simulated Spectrum v10.1.0.vi"() -> ("Simulated Spectrum"=w284:cluster{i32[], dbl[]}[])
                                }
                                }
                                n125 = local read "Target Position"() -> (w251:T9)
                                n126 = Index Array(array=w245, index=0 ("Index")) -> (element=w244:T15)
                                n127 = call "Mapping Merge Live Data.vi"("New Spectrum"=w244, "Target Position"=w251, "X in (1D)"=w259, "Y in (1D)"=w258, "L in (2D)"=w257, "I in (2D)"=w256) -> ("Live Data"=w250:dbl[][], "X out (1D)"=w253:dbl[], "Y out (1D)"=w252:dbl[], "L out (2D)"=w254:dbl[][], "I out (2D)"=w255:dbl[][])  [unwired: 5 in]
                                n128 = invoke class="VI Interface Type 0" method="Ctrl Val.Set"(reference=w261, "Control Name"="LiveData" ("Elementname"), "Value"=w250) -> ()  [unwired: 2 in, 5 out]
                                n129 = local write "Live Data"(w250) -> ()
                              }
                            }
                          }
                          frame #3 {
                            # "set new X"
                            n130 = Increment(x=w295) -> (x+1=w294:i32)
                            n131 = local read "Start"() -> (w288:bool)
                            n132 = Equal?(x=w293, y=w294) -> (x = y?=w285:bool)
                            n133 = Not(x=w288) -> (.not. x?=w287:bool)
                            n134 = Or(x=w285, y=w287) -> (x .or. y?=w286:bool)
                            n135 = case shown="False" w286 {
                              tunnel: w292 -> [w299 w308]
                              tunnel: [w298 w308] -> w289
                              tunnel: w291 -> [w297 _]
                              tunnel: w290 -> [w296 _]
                              frame False {
                                n136 = Unbundle By Name(w299) -> ("Drive X Set"=w300:dbl)
                                n137 = case shown="False" w297 {
                                tunnel: w300 -> [w304 w306]
                                tunnel: [w303 w307] -> w301
                                tunnel: w296 -> [w302 w305]
                                frame False {
                                n138 = Subtract(x=w304, y=w302) -> (x-y=w303:dbl)
                                }
                                frame True {
                                n139 = Add(x=w306, y=w305) -> (x+y=w307:dbl)
                                }
                                }
                                n140 = Bundle By Name(cluster=w299, "Drive X Set"=w301) -> (w298:T13)
                              }
                              frame True {
                              }
                            }
                            n141 = local write "Target Position"(w289) -> ()
                          }
                          frame #4 {
                            n142 = Tick Count (ms)() -> (millisecond timer value=w313:u32)
                            n143 = Subtract(x=w313, y=w312) -> (x-y=w315:u32)
                            n144 = Divide(x=w315, y=u32 1000) -> (x/y=w310:dbl)
                            n145 = Build Array (concatenate)(w311, w310) -> (w309:dbl[])
                          }
                        }
                        n146 = local read "Start"() -> (w177:bool)
                      }
                    }
                    frame #1 {
                      # "set new Y"
                      n147 = Increment(x=w327) -> (x+1=w326:i32)
                      n148 = local read "Start"() -> (w317:bool)
                      n149 = Equal?(x=w325, y=w326) -> (x = y?=w319:bool)
                      n150 = local read "Simulate Drive"() -> (w320:bool)
                      n151 = Not(x=w317) -> (.not. x?=w318:bool)
                      n152 = Or(x=w319, y=w318) -> (x .or. y?=w316:bool)
                      n153 = case shown="False" w316 {
                        tunnel: w323 -> [w345 w346]
                        tunnel: [w344 w346] -> w321
                        tunnel: w324 -> [w341 _]
                        frame False {
                          n154 = Unbundle By Name(w345) -> ("Drive Y Set"=w342:dbl)
                          n155 = Add(x=w341, y=w342) -> (x+y=w343:dbl)
                          n156 = Bundle By Name(cluster=w345, "Drive Y Set"=w343) -> (w344:T13)
                        }
                        frame True {
                        }
                      }
                      n157 = case shown="False" w320 {
                        tunnel: w322 -> [w331 _]
                        tunnel: w321 -> [w330 _]
                        frame False {
                          n158 = local read "Current Position"() -> (w329:T4)
                          n159 = Unbundle By Name(w329) -> ("Voltages.Drive Y Voltage"=w328:dbl)
                          n160 = flat-sequence {
                            tunnel: w331 -> [w334]
                            tunnel: w330 -> [w335]
                            tunnel: w328 -> [w336]
                            tunnel: [w334] -> w333
                            tunnel: [w340] -> w332
                            tunnel: w333 -> [w339]
                            frame #0 {
                              n161 = control-ref of="Objective Running"() -> (w338:refnum<vi>)
                              n162 = call "ESA-C Move Axis To.vi"("Drive Connection Settings"=w334, "Axis"=2, "Current Voltage (V)"=w336, "Drive New Abs. Positions"=w335, "Running"=w338) -> ()  [unwired: 2 in]
                            }
                            frame #1 {
                              n163 = call "ESA-C Get Values.vi"("Drive Connection Settings"=w339) -> ("Drive Current Values"=w340:T4)
                            }
                          }
                          n164 = local write "Current Position"(w332) -> ()
                        }
                        frame True {
                        }
                      }
                      n165 = local write "Target Position"(w321) -> ()
                    }
                  }
                  n166 = local read "Start"() -> (w120:bool)
                }
              }
              frame #2 {
                # "conclude measurement"
                n167 = flat-sequence {
                  tunnel: w348 -> [w351]
                  tunnel: w347 -> [w350]
                  tunnel: w349 -> [w375]
                  frame #0 {
                    # "save data"
                    n168 = local read "CCD3500 Temperature"() -> (w358:dbl)
                    n169 = local read "ITC503 Current Values"() -> (w360:T3)
                    n170 = local read "iHR Current Values"() -> (w359:T5)
                    n171 = local read "Mapping Params"() -> (w354:T10)
                    n172 = local read "Spectra Params"() -> (w355:T6)
                    n173 = local read "Live Data"() -> (w353:dbl[][])
                    n174 = call "Mapping Merge Real Positions.vi"("Live Data In"=w353, "X in (1D)"=w351, "Y in (1D)"=w350) -> ("Live Data Out"=w352:dbl[][])  [unwired: 12 in]
                    "Full Data" <- w352
                    n175 = call "Export_mappingFileName.vi"("ITC503 Current Values"=w360, "iHR Current Values"=w359, "Spectra Settings"=w355, "Mapping Parameters"=w354, "CCD3500 Temperature"=w358) -> ("Filename"=w356:string)
                    "Filename" <- w356
                    n176 = call "Export_2DtoTxt v10.2.0.vi"("Data (2D)"=w352, "Export Type"="Mapping", "Filename"=w356) -> ()  [unwired: 3 in]
                  }
                  frame #1 {
                    # "go to start"
                    n177 = local read "Drive Settings"() -> (w361:T2)
                    n178 = local read "Simulate Drive"() -> (w362:bool)
                    n179 = case shown="False" w362 {
                      tunnel: w361 -> [w364 _]
                      frame False {
                        n180 = stacked-sequence {
                          tunnel: w364 -> [w369 w373]
                          frame #0 {
                            n181 = local read "Mapping Params"() -> (w367:T10)
                            n182 = Unbundle By Name(w367) -> ("X Start Position"=w365:dbl, "Y Start Position"=w366:dbl)
                            n183 = local read "Target Position"() -> (w371:T9)
                            n184 = Bundle By Name(cluster=w371, "Drive X Set"=w365, "Drive Y Set"=w366) -> (w368:T9)
                            n185 = control-ref of="Objective Running"() -> (w370:refnum<vi>)
                            n186 = call "ESA-C Move Absolute.vi"("Running"=w370, "Drive New Abs. Positions"=w368, "Drive Connection Settings"=w369) -> ()  [unwired: 2 in]
                            n187 = local write "Target Position"(w368) -> ()
                          }
                          frame #1 {
                            n188 = call "ESA-C Get Values.vi"("Drive Connection Settings"=w373) -> ("Drive Current Values"=w372:T4)
                            n189 = local write "Current Position"(w372) -> ()
                          }
                        }
                        n190 = property on="Measuring" class="Bool (strict)"("BoolText.Text"="Homing...." ("Boolescher Text.Text")) -> ()  [unwired: 2 in, 2 out]
                      }
                      frame True {
                      }
                    }
                  }
                  frame #2 {
                    # "reset indicators"
                    n191 = case shown="False" w375 {
                      frame False {
                        n192 = call "Video Close.vi"() -> ()  [unwired: 11 in, 1 out]
                      }
                      frame True {
                      }
                    }
                    n193 = local write "Start"(FALSE ("Start")) -> ()
                    n194 = local write "CCD3000 Current Rep."("0/0" ("CCD3000 Current Rep.")) -> ()
                    n195 = property on="Measuring" class="Bool (strict)"("BoolText.Text"="" ("Boolescher Text.Text")) -> ()  [unwired: 2 in, 2 out]
                    n196 = property on="Measuring" class="Bool (strict)"("Blinking"=FALSE ("Measuring")) -> ()  [unwired: 2 in, 2 out]
                  }
                }
              }
            }
          }
        }
        n197 = local read "Exit"() -> (w34:bool)
      }
    }
    frame #2 {
      n198 = invoke class="VI Interface Type 0" method="Ctrl Val.Set"(reference=w379, "Control Name"="Exit" ("Elementname"), "Value"=TRUE) -> ()  [unwired: 2 in, 5 out]
      n199 = flat-sequence {
        frame #0 {
          # "return to center"
          n200 = local read "Simulate Drive"() -> (w382:bool)
          n201 = case shown="False" w382 {
            frame False {
              w388 = 10.0 ("Drive X Set")
              n202 = local read "Z Position"() -> (w387:dbl)
              n203 = local read "Target Position"() -> (w386:T9)
              n204 = local read "Drive Settings"() -> (w385:T2)
              n205 = Bundle By Name(cluster=w386, "Drive X Set"=w388, "Drive Y Set"=w388, "Drive Z Set"=w387) -> (w384:T9)
              n206 = control-ref of="Objective Running"() -> (w383:refnum<vi>)
              n207 = call "ESA-C Move Absolute.vi"("Running"=w383, "Drive New Abs. Positions"=w384, "Drive Connection Settings"=w385) -> ()  [unwired: 2 in]
            }
            frame True {
            }
          }
        }
        frame #1 {
          # "reset and close"
          n208 = control-ref of="Dieses VI"() -> (w389:refnum<vi>)
          n209 = invoke class="VI" method="Default Vals.Reinit All"(reference=w389) -> (reference out=w391:refnum<vi>)  [unwired: 2 in, 2 out]
          n210 = property on="Measuring" class="Bool (strict)"("BoolText.Text"="" ("Boolescher Text.Text")) -> ()  [unwired: 2 in, 2 out]
          n211 = property class="App"() -> ("App.Kind"=w390:T16)  [unwired: 2 in, 2 out]
          n212 = case shown="\"Development System\"" w390 {
            tunnel: w391 -> [w393 _]
            frame "invalid app kind", Default {
              n213 = invoke on="Invoke Node" class="VI" method="FP.Close"(reference=w393) -> ()  [unwired: 2 in, 3 out]
            }
            frame "Development System" {
            }
          }
        }
      }
    }
  }
